vi "Query Connection Type.vi"(8 "error in (no error)":errorcluster, 11 "VISA resource name":refnum<visa-resource-name>) -> (0 "error out":errorcluster, 2 "Type":enum16{"Other", "TCPIP"}(ring), 3 "VISA resource name out":refnum<visa-resource-name>)   [LabVIEW 2015, in "LeCroy Wave Series.lvlib"]
doc: "This VI returns the type of connection."
uses:
  <instrlib>/LeCroy Wave Series/LeCroy Wave Series.lvlib
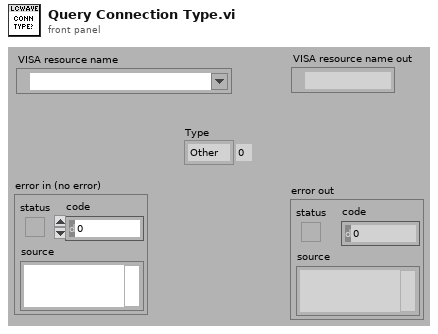
[diagram p1: front panel]
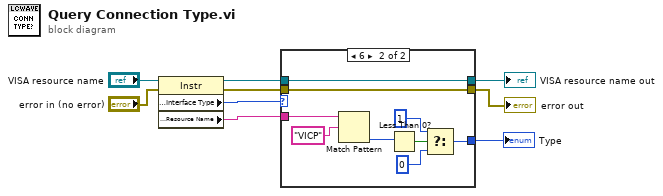
[diagram p0: block diagram]
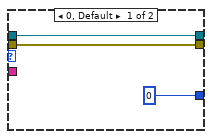
[diagram p2: hidden frame]
diagram:
  n1 = property on="Property Node" class="Instr"(reference="VISA resource name", error in="error in (no error)") -> (reference out=w8:refnum<visa-resource-name>, error out=w7:errorcluster, "Interface Information:Interface Type"=w9:u16, "General Settings:Resource Name"=w1:string)
  n2 = case shown="6" w9 {
    tunnel: w8 -> [w12 w21]
    tunnel: w7 -> [w11 w20]
    tunnel: [w12 w21] -> w6
    tunnel: [w11 w20] -> w5
    tunnel: [0 w15] -> w4
    tunnel: w1 -> [_ w19]
    frame 0, Default {
    }
    frame 6 {
      n3 = Match Pattern(string=w19, regular expression="VICP" ("search string")) -> (offset past match=w13:i32)  [unwired: 1 in, 3 out]
      n4 = Less Than 0?(x=w13) -> (x < 0?=w17:bool)
      n5 = Select(t=1 ("y"), s=w17, f=0 ("y")) -> (s? t:f=w15:i32)
    }
  }
  "VISA resource name out" <- w6
  "error out" <- w5
  "Type" <- w4
